vi "Check if 0.vi"(1 "Axes Magnitudes":cluster{"X":dbl, "Y":dbl, "Z":dbl}) -> (0 "result":bool)   [LabVIEW 2016, in "Huskie Swerve.lvlib"]
uses:
  Huskie Swerve.lvlib
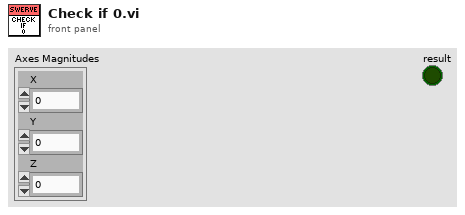
[diagram p1: front panel]
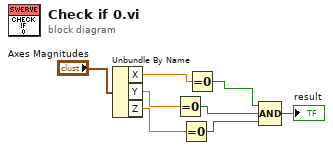
[diagram p0: block diagram]
diagram:
  n1 = Unbundle By Name("Axes Magnitudes") -> ("X"=w4:dbl, "Y"=w3:dbl, "Z"=w2:dbl)
  n2 = Equal To 0?(x=w3) -> (x = 0?=w6:bool)
  n3 = Equal To 0?(x=w2) -> (x = 0?=w7:bool)
  n4 = Equal To 0?(x=w4) -> (x = 0?=w5:bool)
  n5 = Compound Arithmetic op=AND(w5, w6, w7) -> (→"result":bool)
